vi "Laurel Send Receive.vi"(0 "TCP Network Connection in":refnum<k5>, 2 "Serial VISA":refnum<visa-resource-name>, 5 "Laurel Serial Commands":T2, 9 "Individual Byte Count":i32=8, 11 "error in (no error)":errorcluster, 12 "All Items Byte Count (Flow Rate)":i32=17, 13 "Connection Type":T1) -> (1 "Single Item":dbl, 3 "Output String":string="0000.00 0004.71", 4 "TCP Network Connection out":refnum<k5>, 6 "Flow Rate (Item 1)":dbl, 8 "VISA resource name 2":refnum<visa-resource-name>, 10 "Gallons (Item 2)":dbl, 14 "return count":i32, 15 "error out":errorcluster)   [LabVIEW 2016]
uses:
  Type Definitions/Laurel Serial Commands.ctl
  Type Definitions/Laurel Connection Type.ctl
  <vilib>/Utility/error.llb/whitespace.ctl
panel:
  out "Send Command out":string
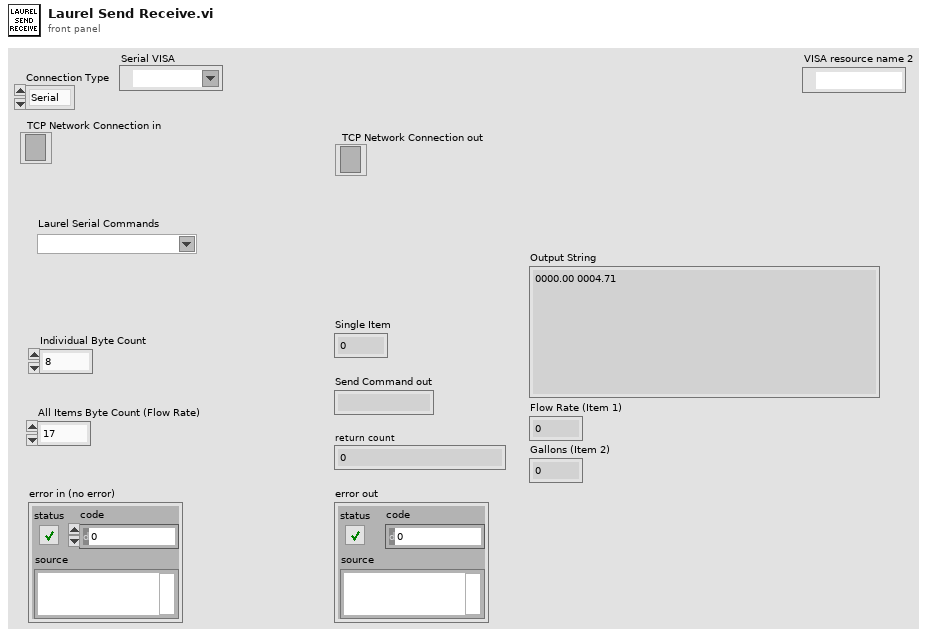
[diagram p1: front panel]
types:
  T1 = typedef "Laurel Connection Type.ctl" = enum16{"Serial", "TCP"}
  T2 = typedef "Laurel Serial Commands.ctl" = string
  T3 = typedef "whitespace.ctl" = u16
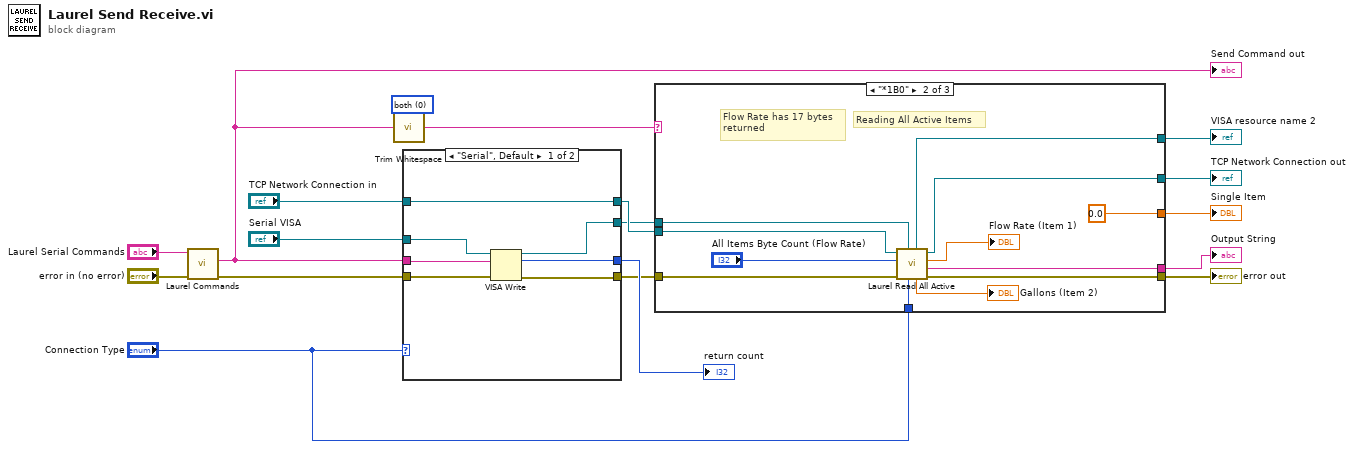
[diagram p0: block diagram]
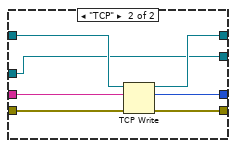
[diagram p2: hidden frame]
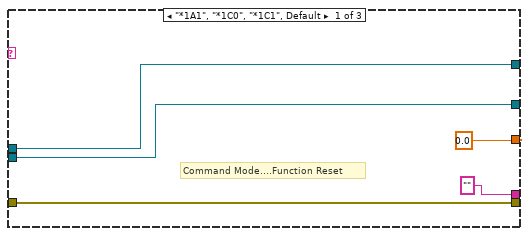
[diagram p3: hidden frame]
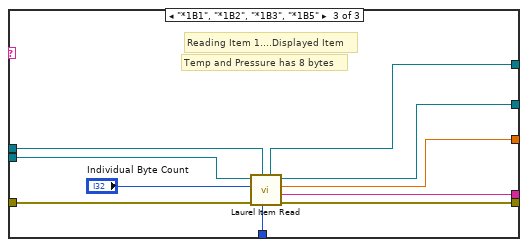
[diagram p4: hidden frame]
diagram:
  w1 = T3 0 items=["both", "start of string", "end of string"] ("location (both)")
  n1 = call "Laurel Commands.vi"("Error In"="error in (no error)", "Laurel Serial Commands"="Laurel Serial Commands") -> ("Error Out"=w11:errorcluster, "Send Command out"=w3:string)  [unwired: 8 in]
  "Send Command out" <- w3
  n2 = call <vilib>:"Trim Whitespace.vi"("string"=w3, "location (both)"=w1) -> ("trimmed string"=w2:string)
  n3 = case shown="\"Serial\", Default" "Connection Type" {
    tunnel: [w21 w32] -> w18
    tunnel: [w24 w31] -> w15
    tunnel: w11 -> [w25 w30]
    tunnel: [w19 w29] -> w10
    tunnel: w3 -> [w23 w28]
    tunnel: [w22 w26] -> w5
    tunnel: "Serial VISA" -> [w20 w26]
    tunnel: "TCP Network Connection in" -> [w19 w27]
    frame "Serial", Default {
      n4 = VISA Write(VISA resource name=w20, write buffer=w23, error in (no error)=w25) -> (VISA resource name out=w22:refnum<visa-resource-name>, return count=w21:u32, error out=w24:errorcluster)
    }
    frame "TCP" {
      n5 = TCP Write(connection ID=w27, data in=w28, error in (no error)=w30) -> (connection ID out=w29:refnum<k5>, bytes written=w32:i32, error out=w31:errorcluster)  [unwired: 1 in]
    }
  }
  "return count" <- w18
  n6 = case shown="\"*1B0\"" w2 {
    tunnel: [w34 w49 w54] -> w14
    tunnel: [0.0 0.0 w59] -> w17
    tunnel: ["" ("read buffer") w44 w58] -> w13
    tunnel: w10 -> [w35 w47 w57]
    tunnel: w15 -> [w34 w46 w56]
    tunnel: [w35 w48 w53] -> w16
    tunnel: "Connection Type" -> [_ w41 w52]
    tunnel: w5 -> [w33 w39 w51]
    tunnel: [w33 w38 w50] -> w4
    frame "*1A1", "*1C0", "*1C1", Default {
      # "Command Mode....Function Reset"
    }
    frame "*1B0" {
      # "Reading All Active Items"
      # "Flow Rate has 17 bytes \nreturned"
      n7 = call "Laurel Read All Active.vi"("Connection Type"=w41, "VISA resource name"=w39, "error in (no error)"=w46, "byte count in"="All Items Byte Count (Flow Rate)", "TCP Network Connection in"=w47) -> ("error out"=w49:errorcluster, "trimmed string"=w44:string, "Flow Rate (Item 1)"=→"Flow Rate (Item 1)":dbl, "TCP Network Connection out"=w48:refnum<k5>, "Gallons (Item 2)"=→"Gallons (Item 2)":dbl, "VISA resource name 2"=w38:refnum<visa-resource-name>)  [unwired: 1 in]
    }
    frame "*1B1", "*1B2", "*1B3", "*1B5" {
      # "Reading Item 1....Displayed Item"
      # "Temp and Pressure has 8 bytes"
      n8 = call "Laurel Item Read.vi"("Connection Type"=w52, "VISA resource name"=w51, "error in (no error)"=w56, "byte count"="Individual Byte Count", "TCP Network Connection in"=w57) -> ("error out"=w54:errorcluster, "trimmed string"=w58:string, "Numeric"=w59:dbl, "TCP Network Connection out"=w53:refnum<k5>, "VISA resource name 2"=w50:refnum<visa-resource-name>)  [unwired: 2 in]
    }
  }
  "Single Item" <- w17
  "TCP Network Connection out" <- w16
  "error out" <- w14
  "Output String" <- w13
  "VISA resource name 2" <- w4
